vi "utility.ReadFrame.vi"(6 "Frame长度":u32, 7 "timeout(ms)":u32=9000 caption="超时（ms）", 8 "error in (no error)":errorcluster caption="错误输入（无错误）", 10 "Para":cluster{u8[][]}[](array[cluster]), 11 "FrameReader":refnum<visa-resource-name>="COM5") -> (0 "error out":errorcluster={"status"=FALSE, "code"=1073676294, "source"="Lib_UEL.ATE.lvlib:Lib_2Voice.lvlib:2Voice.FRAME_RD.vi->Lib_UEL.ATE.lvlib:Lib_App.lvlib:utility.ReadFrame.vi中的VISA读取"} caption="错误输出", 3 "OK?":bool=TRUE)   [LabVIEW 2012, in "Lib_UEL.ATE.lvlib" / "Lib_App.lvlib"]
uses:
  Lib_App.lvlib
  2Voice/Lib_2Voice.lvlib
panel:
  out "OK? 2":bool
  out "Process":bool[](array[boolean])
  in  "Test Frame":string="<---\r\n"
  # "V1.0 初始版本。\nV1.1 增加多选一判定。\n- 每个按键可以使用多个备用Frame，只要一个正确即可。"
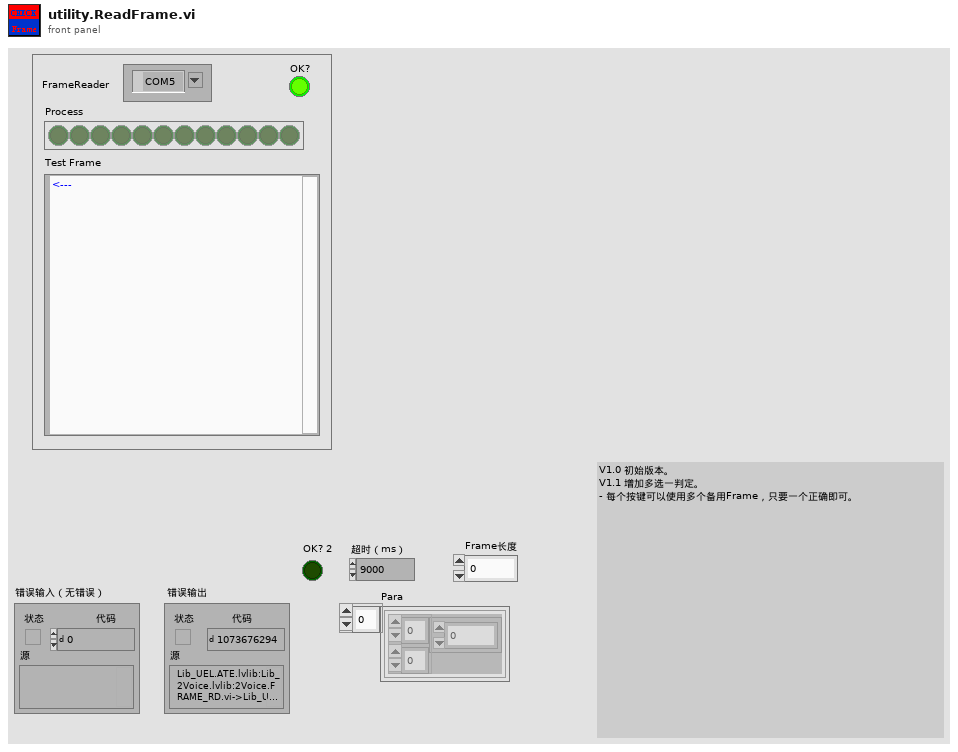
[diagram p1: front panel]
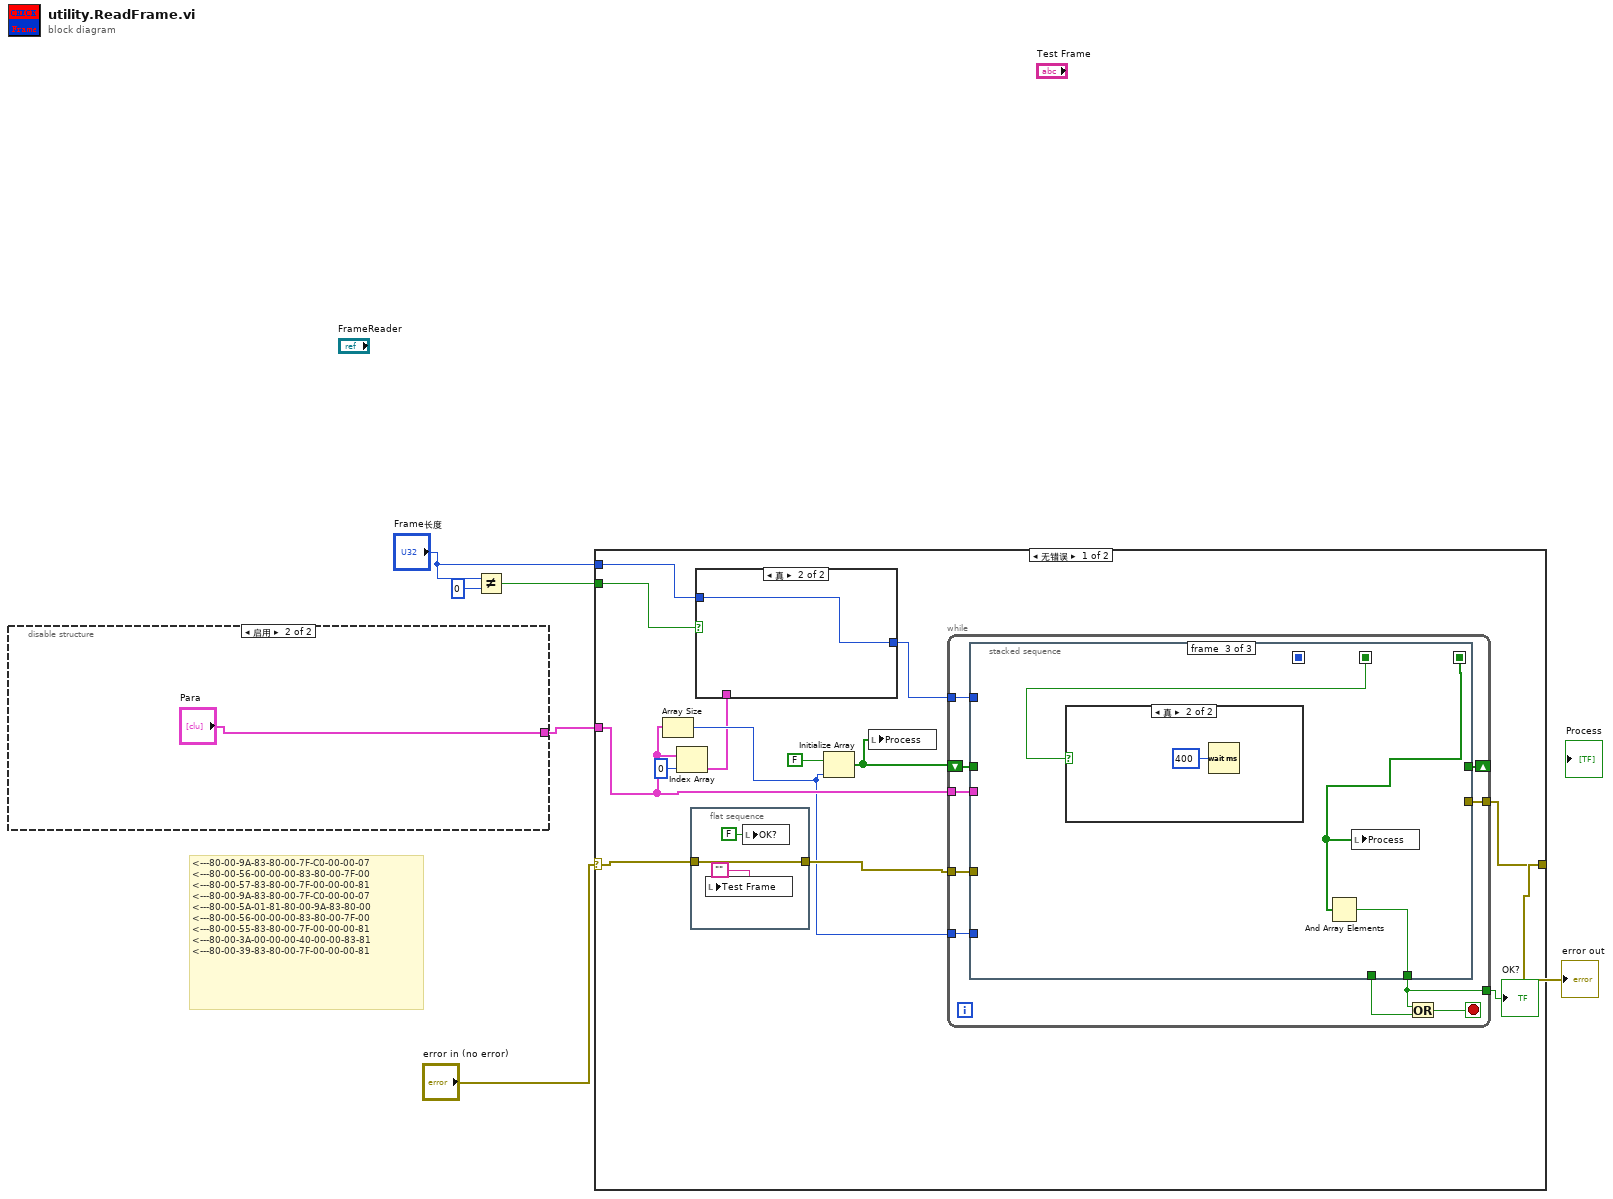
[diagram p0: block diagram]
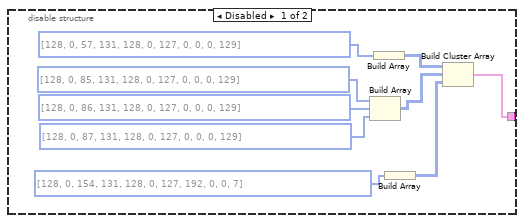
[diagram p2: hidden frame]
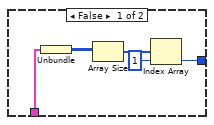
[diagram p3: hidden frame]
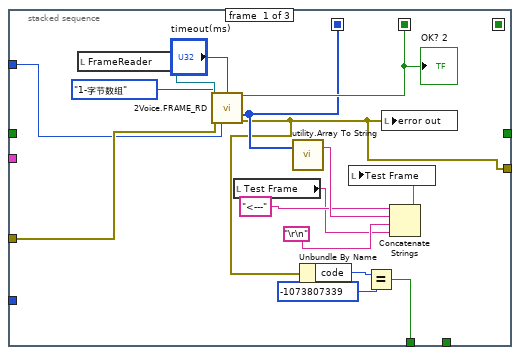
[diagram p4: hidden frame]
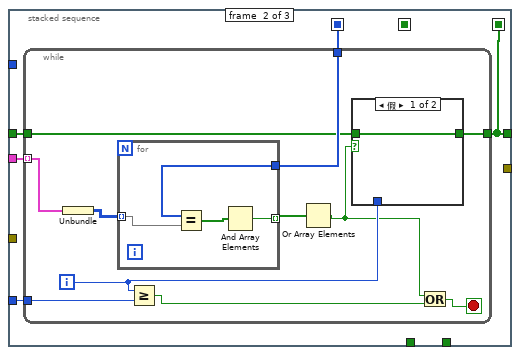
[diagram p5: hidden frame]
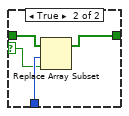
[diagram p6: hidden frame]
diagram:
  # "<---80-00-9A-83-80-00-7F-C0-00-00-07\n<---80-00-56-00-00-00-83-80-00-7F-00\n<---80-00-57-83-80-00-7F-00-00-00-81\n<---80-00-9A-83-80-00-7F-C0-00-00-07\n<---80-00-5A-01-81-80-00-9A-83-80-00\n<---80-00-56-00-00-00-83-80-00-7F-00\n<---80-00-55-83-80-00-7F-00-00-00-81\n<---80-00-3A-00-00-00-40-00-00-83-81\n<---80-00-39-83-80-00-7F-00-00-00-81"
  n1 = disable-structure shown="启用" {
    disable-tunnel: [w7 "Para"] -> w1
    frame Disabled {
      n2 = Build Array(u8[] [128, 0, 85, 131, 128, 0, 127, 0, 0, 0, 129] ("Para"), u8[] [128, 0, 86, 131, 128, 0, 127, 0, 0, 0, 129] ("Para"), u8[] [128, 0, 87, 131, 128, 0, 127, 0, 0, 0, 129] ("Para")) -> (w9:u8[][])
      n3 = Build Array(u8[] [128, 0, 57, 131, 128, 0, 127, 0, 0, 0, 129] ("Para")) -> (w10:u8[][])
      n4 = Build Array(u8[] [128, 0, 154, 131, 128, 0, 127, 192, 0, 0, 7] ("Para")) -> (w8:u8[][])
      n5 = Build Cluster Array(w10, w9, w8) -> (w7:cluster{u8[][]}[])
    }
    frame Enabled {
    }
  }
  n6 = Not Equal?(x="Frame长度", y=u32 0) -> (x != y?=w3:bool)
  n7 = case shown="无错误" "error in (no error)" {
    selector: "error in (no error)" -> [w25 w94]
    tunnel: [w28 w94] -> w5
    tunnel: w1 -> [w23 _]
    tunnel: w3 -> [w18 _]
    tunnel: "Frame长度" -> [w17 _]
    frame No Error {
      n8 = Array Size(array=w23) -> (size(s)=w22:i32)
      n9 = Index Array(array=w23, index=0 ("索引")) -> (element=w21:cluster{u8[][]})
      n10 = flat-sequence {
        tunnel: [w37] -> w26
        tunnel: w25 -> [w37]
        frame #0 {
          n11 = local write "Test Frame"("") -> ()
          n12 = local write "OK?"(FALSE ("OK?")) -> ()
        }
      }
      n13 = case shown="真" w18 {
        tunnel: w21 -> [w34 _]
        tunnel: [w30 w35] -> w19
        tunnel: w17 -> [_ w35]
        frame False {
          n14 = Unbundle(w34) -> (w33:u8[][])
          n15 = Array Size(array=w33) -> (size(s)=w32:i32[])
          n16 = Index Array(array=w32, index=1 ("索引")) -> (element=w30:i32)
        }
        frame True {
        }
      }
      n17 = Initialize Array(FALSE, w22) -> (w24:bool[])
      n18 = local write "Process"(w24) -> ()
      n19 = while {
        tunnel: w23 -> [w48]
        shift-right: [w43] -> _
        shift-left: w24 -> [w44]
        tunnel: w22 -> [w45]
        tunnel: w26 -> [w42]
        tunnel: [w41] -> w28
        tunnel: [w40] -> w27
        tunnel: w19 -> [w39]
        stop <- w46 stop-if-true
        n20 = stacked-sequence {
          seq-local: [w59 _ _] -> [_ _ w90]
          seq-local: [w58 _ _] -> [_ w68 _]
          seq-local: [_ w66 _] -> [_ _ w91]
          tunnel: w48 -> [_ w65 _]
          tunnel: [w49 _ _] -> w47
          tunnel: w45 -> [_ w69 _]
          tunnel: w44 -> [_ w67 _]
          tunnel: [_ w66 _] -> w43
          tunnel: [_ _ w92] -> w40
          tunnel: w42 -> [w55 _ _]
          tunnel: [w54 _ _] -> w41
          tunnel: w39 -> [w50 _ _]
          frame #0 {
            n21 = local read "FrameReader"() -> (w64:refnum<visa-resource-name>)
            n22 = call "2Voice.FRAME_RD.vi"("VISA resource name"=w64, "timeout(ms)"="timeout(ms)", "ReadMode"=enum16{"0-字符串", "1-字节数组"}."1-字节数组", "error in (no error)"=w55, "字节总数"=w50) -> ("OK?"=w59:bool, "读出字节数组"=w58:u8[], "error out"=w54:errorcluster)  [unwired: 6 in, 2 out]
            "OK? 2" <- w59
            n23 = local read "Test Frame"() -> (w51:string)
            n24 = call "utility.Array To String.vi"("无符号字节数组"=w58) -> ("命令输出(字符串)"=w61:string)  [unwired: 1 in, 1 out]
            n25 = Unbundle By Name(w54) -> ("code"=w57:i32)
            n26 = Equal?(x=w57, y=-1073807339) -> (x = y?=w49:bool)
            n27 = local write "error out"(w54) -> ()
            n28 = Concatenate Strings("<---" ("字符串"), w61, "\r\n", w51) -> (w63:string)
            n29 = local write "Test Frame"(w63) -> ()
          }
          frame #1 {
            n30 = while {
              tunnel: w69 -> [w80]
              tunnel: w68 -> [w79]
              tunnel: w67 -> [w75]
              tunnel: [w74] -> w66
              tunnel: w65 -> [w71] mode=indexing
              i -> [w76]
              stop <- w78 stop-if-true
              n31 = Unbundle(w71) -> (w70:u8[][])
              n32 = for {
                tunnel: w79 -> [w84]
                tunnel: [w82] -> w73 mode=indexing
                tunnel: w70 -> [w81] mode=indexing
                n33 = Equal?(x=w84, y=w81) -> (x = y?=w83:bool[])
                n34 = And Array Elements(Boolean array=w83) -> (logical AND=w82:bool)
              }
              n35 = Greater Or Equal?(x=w76, y=w80) -> (x >= y?=w77:bool)
              n36 = Or Array Elements(Boolean array=w73) -> (logical OR=w72:bool)
              n37 = case shown="假" w72 {
                selector: w72 -> [_ w87]
                tunnel: w76 -> [_ w89]
                tunnel: w75 -> [w85 w88]
                tunnel: [w85 w86] -> w74
                frame False {
                }
                frame True {
                  n38 = Replace Array Subset(array=w88, new element=w87, index=w89) -> (w86:bool[])
                }
              }
              n39 = Or(x=w72, y=w77) -> (x .or. y?=w78:bool)
            }
          }
          frame #2 {
            n40 = case shown="真" w90 {
              frame False {
              }
              frame True {
                n41 = Wait (ms)(milliseconds to wait=u32 400 ("等待时间（毫秒）")) -> ()  [unwired: 1 out]
              }
            }
            n42 = And Array Elements(Boolean array=w91) -> (logical AND=w92:bool)
            n43 = local write "Process"(w91) -> ()
          }
        }
        n44 = Or(x=w40, y=w47) -> (x .or. y?=w46:bool)
      }
      "OK?" <- w27
    }
    frame Error {
    }
  }
  "error out" <- w5
